vi "Clean Up Name from Member.vi"(1 "Name Input":string) -> (0 "Clean Name Output":string)   [LabVIEW 2020]
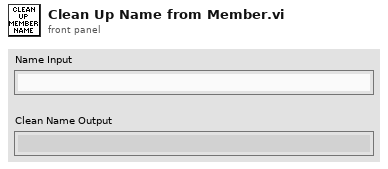
[diagram p1: front panel]
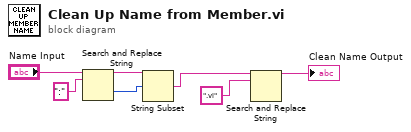
[diagram p0: block diagram]
diagram:
  n1 = Search and Replace String(input string="Name Input", search string=":") -> (result string=w3:string, offset past replacement=w1:i32)  [unwired: 6 in, 2 out]
  n2 = String Subset(string=w3, offset (0)=w1) -> (substring=w2:string)  [unwired: 1 in]
  n3 = Search and Replace String(input string=w2, search string=".vi") -> (result string=→"Clean Name Output":string)  [unwired: 6 in, 3 out]
